vi "AES N Teeth M Missing Generation.vi"(4 "NTeeth.TDC Offset":fxp<+/-,61,10>, 5 "NTeeth.Reset":bool, 6 "NTeeth.Missing Teeth Offset":fxp<+,61,10>, 7 "NTeeth.TopDeadCenter High?":bool=TRUE, 8 "NTeeth.Missing Teeth Gap":fxp<+,61,10>, 9 "NTeeth.Degrees Low Pulse":fxp<+,60,9>, 10 "NTeeth.Degrees High Pulse":fxp<+,60,9>, 11 "Crank or Cyle Angle":fxp<+,61,10>) -> (3 "NTeeth.Digital Output":bool)   [LabVIEW 2010, in "AES.lvlib" / "AES FPGA.lvlib"]
doc: "This IP generates a digital signal to simulate N teeth with M missing according to some setting inputs. This is most commonly used for Crank simulation. This IP emulates a signal that has a certain number of teeth with some missing (i.e. 60 teeth & 2 missing). The number of teeth and number of teeth missing can be configured. \n\nThe signal generation IP adds the flexibility of configuring duty cycle of pulses (i.e. degrees high and degrees low), an offset to where the missing teeth are located, and whether top dead center (0 degrees) begins with a low pulse or high pulse. These configurations should not be changed and should be made before the FPGA is told to run.\n\nNOTE: If the gap spans across TDC (0 Degrees) this will not handle it appropriately!"
uses:
  AES FPGA.lvlib
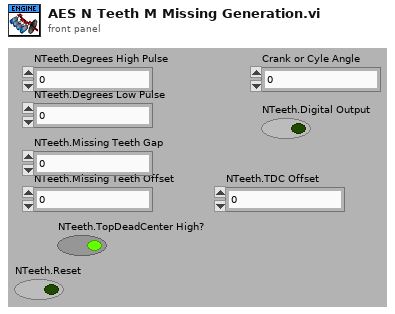
[diagram p1: front panel]
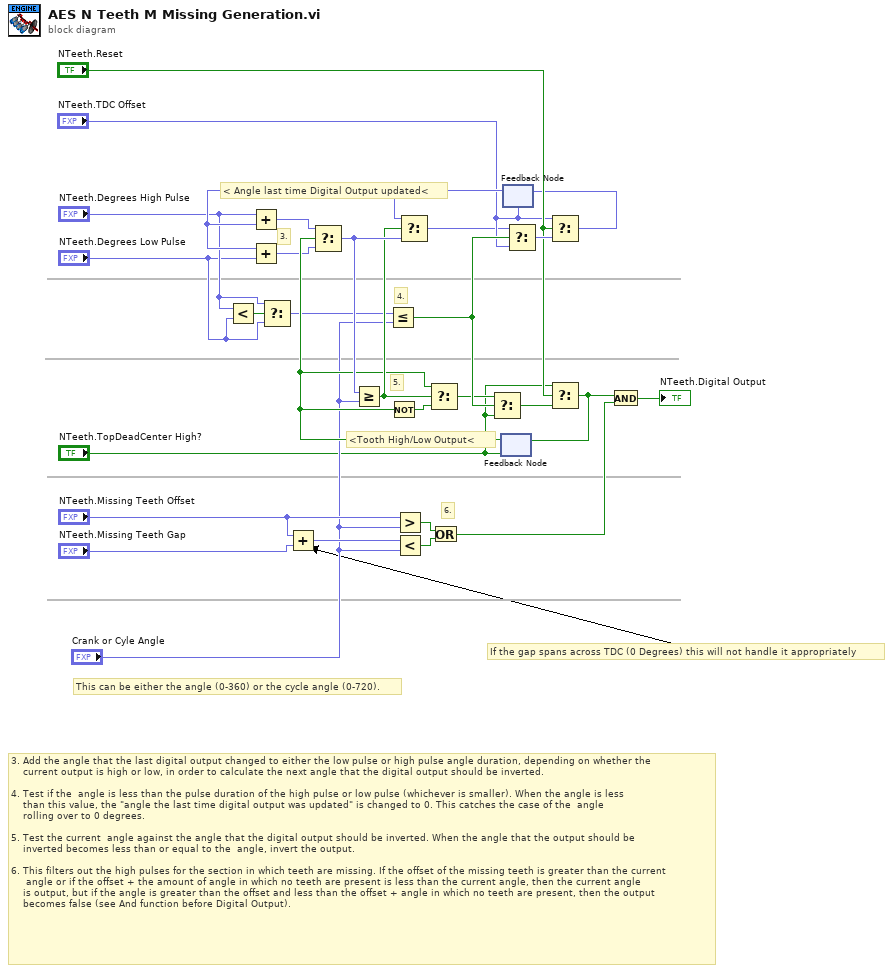
[diagram p0: block diagram]
diagram:
  # "If the gap spans across TDC (0 Degrees) this will not handle it appropriately"
  # "This can be either the angle (0-360) or the cycle angle (0-720)."
  # "6."
  # "<Tooth High/Low Output<"
  # "5."
  # "< Angle last time Digital Output updated<"
  # "4."
  # "3."
  # "3. Add the angle that the last digital output changed to either the low pulse or high pulse angle duration, depending on whether the\n    current output is high or low, in order to calculate the next angle that the digital output should be inverted.\n\n4. Test if the  angle is less than the pulse duration of the high pulse or low pulse (whichever is smaller). When the angle is less\n    than this value, the \"angle the last time digital output was updated\" is changed to 0. This catches the case of the  angle \n    rolling over to 0 degrees.\n\n5. Test the current  angle against the angle that the digital output should be inverted. When the angle that the output should be\n    inverted becomes less than or equal to the  angle, invert the output.\n\n6. This filters out the high pulses for the section in which teeth are missing. If the offset of the missing teeth is greater than the current\n     angle or if the offset + the amount of angle in which no teeth are present is less than the current angle, then the current angle\n    is output, but if the angle is greater than the offset and less than the offset + angle in which no teeth are present, then the output\n    becomes false (see And function before Digital Output)."
  n1 = Less?(x="NTeeth.Degrees High Pulse", y="NTeeth.Degrees Low Pulse") -> (x < y?=w19:bool)
  n2 = Select(t="NTeeth.Degrees High Pulse", s=w19, f="NTeeth.Degrees Low Pulse") -> (s? t:f=w16:fxp<+,60,9>)
  n3 = Add(x="NTeeth.Missing Teeth Offset", y="NTeeth.Missing Teeth Gap") -> (x+y=w15:fxp<+,62,11>)
  n4 = Less Or Equal?(x=w16, y="Crank or Cyle Angle") -> (x <= y?=w28:bool)
  n5 = Greater?(x="NTeeth.Missing Teeth Offset", y="Crank or Cyle Angle") -> (0:w12:bool)
  n6 = Less?(x=w15, y="Crank or Cyle Angle") -> (x < y?=w11:bool)
  n7 = Or(x=w12, y=w11) -> (x .or. y?=w10:bool)
  n8 = feedback #1("NTeeth.TopDeadCenter High?") -> (w22:bool)
  n9 = Not(x=w22) -> (.not. x?=w21:bool)
  n10 = feedback #2("NTeeth.TDC Offset") -> (w25:fxp<+/-,62,11>)
  n11 = Add(x="NTeeth.Degrees High Pulse", y=w25) -> (x+y=w26:fxp<+,61,10>)
  n12 = Add(x=w25, y="NTeeth.Degrees Low Pulse") -> (x+y=w20:fxp<+,61,10>)
  n13 = Select(t=w26, s=w22, f=w20) -> (s? t:f=w24:fxp<+,61,10>)
  n14 = Greater Or Equal?(x=w24, y="Crank or Cyle Angle") -> (x >= y?=w23:bool)
  n15 = Select(t=w25, s=w23, f=w24) -> (s? t:f=w2:fxp<+/-,62,11>)
  n16 = Select(t=w22, s=w23, f=w21) -> (s? t:f=w27:bool)
  n17 = Select(t=w27, s=w28, f="NTeeth.TopDeadCenter High?") -> (s? t:f=w6:bool)
  n18 = Select(t=w2, s=w28, f="NTeeth.TDC Offset") -> (s? t:f=w8:fxp<+/-,62,11>)
  n19 = Select(t="NTeeth.TDC Offset", s="NTeeth.Reset", f=w8) -> (s? t:f=w1:fxp<+/-,62,11>)
  n20 = feedback-in #2(w1) -> ()
  n21 = Select(t="NTeeth.TopDeadCenter High?", s="NTeeth.Reset", f=w6) -> (s? t:f=w7:bool)
  n22 = feedback-in #1(w7) -> ()
  n23 = And(x=w7, y=w10) -> (x .and. y?=→"NTeeth.Digital Output":bool)
